vi "GEN_Time-coded_overlay.vi"(0 "Time-coded overlay refnum in":T1, 5 "Full track array":T2(array[cluster]), 7 "Multiline grouping, samples":i32=100, 9 "Samples full merge, every N":i32=1000, 11 "error in (no error)":errorcluster) -> (4 "Time-coded overlay refnum out":T1, 15 "error out":errorcluster)   [LabVIEW 2018, in "Tracker.lvlib"]
uses:
  Tracker.lvlib
  <vilib>/vision/Image Controls.llb/IMAQ Image.ctl
  Controls/CTL_Color_ramp.ctl
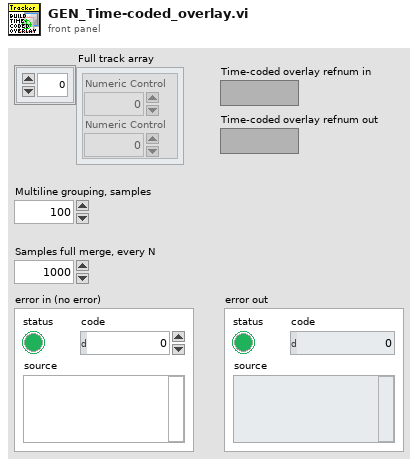
[diagram p1: front panel]
types:
  T1 = typedef "IMAQ Image.ctl" = refnum<image>
  T2 = cluster{"Numeric Control":dbl, "Numeric Control":dbl}[]
  T3 = typedef "Tracker.lvlib/CTL_Color_ramp.ctl" = u32[]
  T4 = cluster{"Numeric Control":dbl, "Numeric Control":dbl}
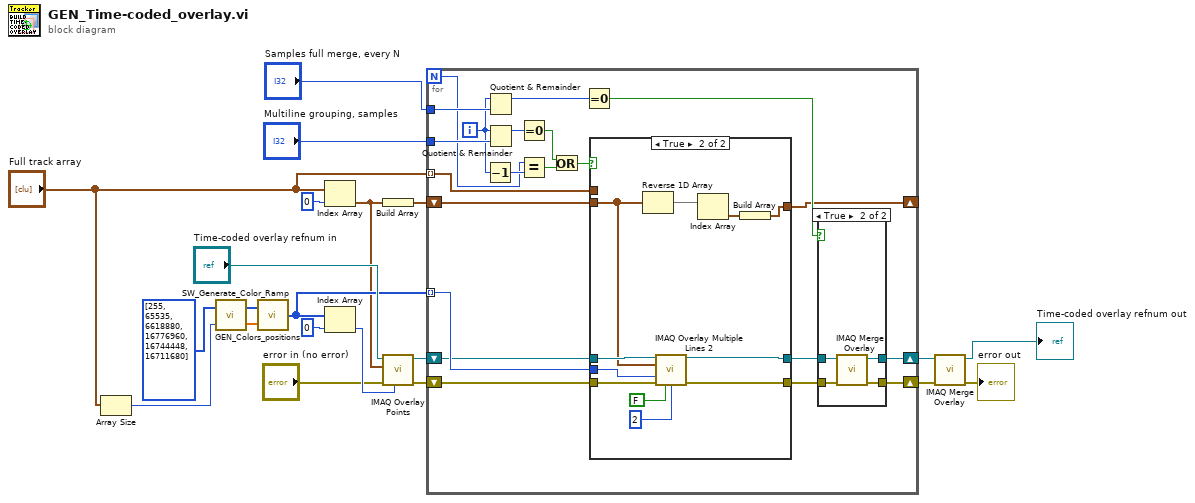
[diagram p0: block diagram]
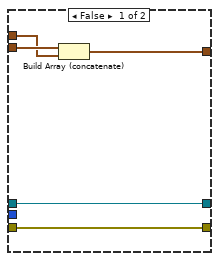
[diagram p2: hidden frame]
diagram:
  n1 = Array Size(array="Full track array") -> (size(s)=w16:i32)
  n2 = call "GEN_Colors_positions.vi"("Highest color position"=w16, "Initial colors ramp array in"=T3 [255, 65535, 6618880, 16776960, 16744448, 16711680] ("Initial colors ramp array")) -> ("Colors positions"=w19:dbl[], "Initial colors ramp array out"=w20:T3)
  n3 = call "SW_Generate_Color_Ramp.vi"("Colors rel. pos."=w19, "Colors array"=w20) -> ("Colors array"=w17:u32[])
  n4 = Index Array(array="Full track array", index=0) -> (element=w8:T4)
  n5 = Index Array(array=w17, index=0) -> (element=w4:u32)
  n6 = Build Array(w8) -> (w9:T2)
  n7 = call "IMAQ Overlay Points"("Color"=w4, "error in (no error)"="error in (no error)", "Point"=w8, "Image"="Time-coded overlay refnum in") -> ("error out"=w1:errorcluster, "Image Out"=w7:T1)  [unwired: 6 in]
  n8 = for {
    N -> [w24]
    shift-right: [w41] -> w10
    shift-left: w7 -> [w35]
    tunnel: "Full track array" -> [w39] mode=indexing
    tunnel: w17 -> [w37] mode=indexing
    shift-right: [w27] -> w13
    shift-left: w1 -> [w30]
    shift-right: [w34] -> _
    shift-left: w9 -> [w38]
    tunnel: "Multiline grouping, samples" -> [w31]
    tunnel: "Samples full merge, every N" -> [w29]
    i -> [w26]
    n9 = Decrement(x=w26) -> (x-1=w25:i32)
    n10 = Quotient & Remainder(x=w26, y=w29) -> (x-y*floor(x/y)=w40:i32)  [unwired: 1 out]
    n11 = Quotient & Remainder(x=w26, y=w31) -> (x-y*floor(x/y)=w33:i32)  [unwired: 1 out]
    n12 = Equal To 0?(x=w33) -> (x = 0?=w32:bool)
    n13 = Equal?(x=w24, y=w25) -> (x = y?=w22:bool)
    n14 = Or(x=w32, y=w22) -> (x .or. y?=w23:bool)
    n15 = Equal To 0?(x=w40) -> (x = 0?=w42:bool)
    n16 = case shown="True" w23 {
      tunnel: w39 -> [w44 _]
      tunnel: w38 -> [w46 w52]
      tunnel: w37 -> [_ w58]
      tunnel: w30 -> [w43 w57]
      tunnel: [w47 w56] -> w36
      tunnel: [w43 w55] -> w28
      tunnel: w35 -> [w47 w54]
      tunnel: [w45 w49] -> w34
      frame False {
        n17 = Build Array (concatenate)(w46, w44) -> (w45:T2)
      }
      frame True {
        n18 = Reverse 1D Array(array=w52) -> (reversed array=w51:T2)
        n19 = call "IMAQ Overlay Multiple Lines 2"("Image"=w54, "Line End Points"=w52, "Color"=w58, "error in (no error)"=w57, "Maintain Width?"=FALSE, "Width"=u32 2) -> ("Image Out"=w56:T1, "error out"=w55:errorcluster)  [unwired: 8 in]
        n20 = Index Array(array=w51) -> (element=w50:T4)  [unwired: 1 in]
        n21 = Build Array(w50) -> (w49:T2)
      }
    }
    n22 = case shown="True" w42 {
      tunnel: w36 -> [w60 w64]
      tunnel: [w60 w63] -> w41
      tunnel: w28 -> [w59 w62]
      tunnel: [w59 w61] -> w27
      frame False {
      }
      frame True {
        n23 = call "IMAQ Merge Overlay"("error in (no error)"=w62, "Image Src"=w64) -> ("error out"=w61:errorcluster, "Image Dst Out"=w63:T1)  [unwired: 8 in]
      }
    }
  }
  n24 = call "IMAQ Merge Overlay"("error in (no error)"=w13, "Image Src"=w10) -> ("error out"=→"error out":errorcluster, "Image Dst Out"=→"Time-coded overlay refnum out":T1)  [unwired: 8 in]
